vi "Count by Status.vi"(10 "Status":T7, 11 "Test Suite Result in":T1) -> (2 "Count":i32, 3 "Test Suite Result out":T1)   [LabVIEW 2020, in "Test Suite Result.lvlib"]
uses:
  Test Suite Result.lvlib
  Test Suite Result.ctl
  Core/Result/Status.ctl
  Case Result/Test Case Result.ctl
  Method Result/Method Result.ctl
  Assertion Result/Assertion Result.ctl
  Assertion Result/Public/TypeDefs/Assertion Type.ctl
  Assertion Result/Public/TypeDefs/Status.ctl
  Case Result/Private/Merge Status.vi
  Case Result/Test Case Result.lvlib
  Assertion Result/Assertion Result.lvlib
  Method Result/Method Result.lvlib
  Core/Result/Result.lvlib
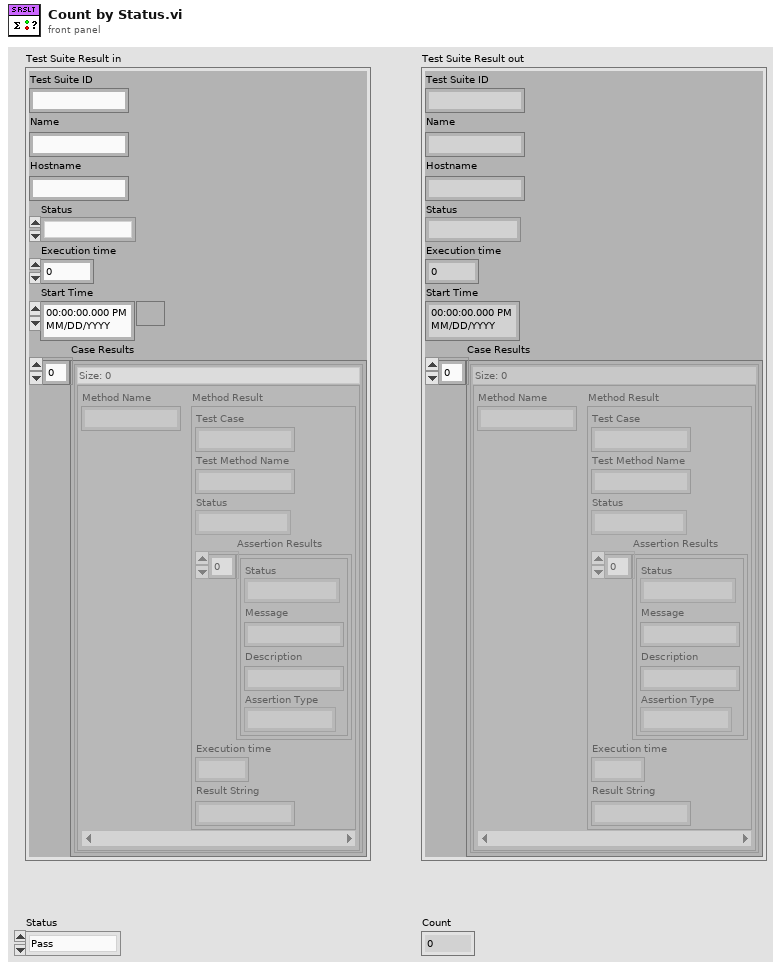
[diagram p1: front panel]
types:
  T1 = typedef "Test Suite Result.lvlib/Test Suite Result.ctl" = cluster{"Test Suite ID":string, "Name":string, "Hostname":string, "Status":T2, "Execution time":dbl, "Start Time":timestamp, "Case Results":T3[]}
  T2 = typedef "Result.lvlib/Status.ctl" = enum16{"", "Passed", "Failed", "Error", "Skipped", "Setup Error", "Broken", "Teardown Error"}
  T3 = typedef "Test Case Result.lvlib/Test Case Result.ctl" = map{string, T4}
  T4 = typedef "Method Result.lvlib/Method Result.ctl" = cluster{"Test Case":string, "Test Method Name":string, "Status":T2, "Assertion Results":T5[], "Execution time":dbl, "Result String":string}
  T5 = typedef "Assertion Result.lvlib/Assertion Result.ctl" = cluster{"Status":T2, "Message":string, "Description":string, "Assertion Type":T6}
  T6 = typedef "Result.lvlib/Assertion Type.ctl" = enum16{"None", "Pass", "Fail", "Skip", "Pass if Equal", "Fail if Equal", "Pass if Error", "Fail if Error", "Pass if", "Fail if"}
  T7 = typedef "Assertion Result.lvlib/Status.ctl" = enum16{"Pass", "Fail", "Error", "Skipped", "Setup Error", "Broken", "Teardown Error"}
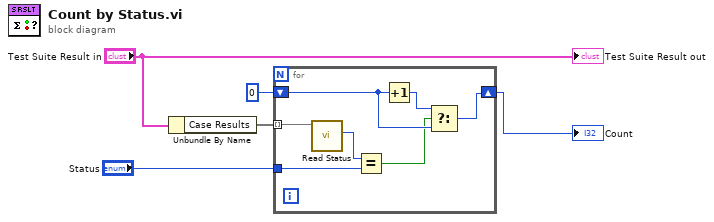
[diagram p0: block diagram]
diagram:
  n1 = Unbundle By Name("Test Suite Result in") -> ("Case Results"=w1:T3[])
  n2 = for {
    tunnel: w1 -> [w12] mode=indexing
    tunnel: "Status" -> [w10]
    shift-right: [w7] -> w5
    shift-left: 0 -> [w8]
    n3 = call "Read Status.vi"("Test Case Result In"=w12) -> ("Status"=w11:T2)  [unwired: 8 in, 2 out]
    n4 = Equal?(x=w11, y=w10) -> (x = y?=w6:bool)
    n5 = Increment(x=w8) -> (x+1=w9:i32)
    n6 = Select(t=w9, s=w6, f=w8) -> (s? t:f=w7:i32)
  }
  "Count" <- w5
  "Test Suite Result out" <- "Test Suite Result in"
